vi "Fit VI window to Largest Dec__ogtk.vi"(4 "error in (no error)":errorcluster, 6 "border spacing (2 px)":i32=2, 7 "VI Ref (calling VI)":refnum<vi>) -> (0 "error out":errorcluster, 3 "dup VI Ref":refnum<vi>)   [LabVIEW 2017]
doc: "This utility will fit (resize and center) a VI (defined by the \"VI Ref\" input) about the largest decoration in that VI. It will add a border defined by border spacing in units of pixels. If there are no decorations found in the VI it is a no-op and will not produce an error. Unfortunately, this VI can not find locked decorations (yet)."
uses:
  <vilib>/Utility/miscctls.llb/LVRectTypeDef.ctl
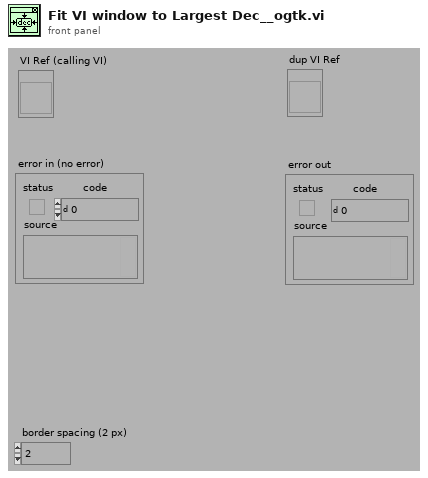
[diagram p1: front panel]
types:
  T1 = typedef "LVRectTypeDef.ctl" = cluster{"Left":i16, "Top":i16, "Right":i16, "Bottom":i16}
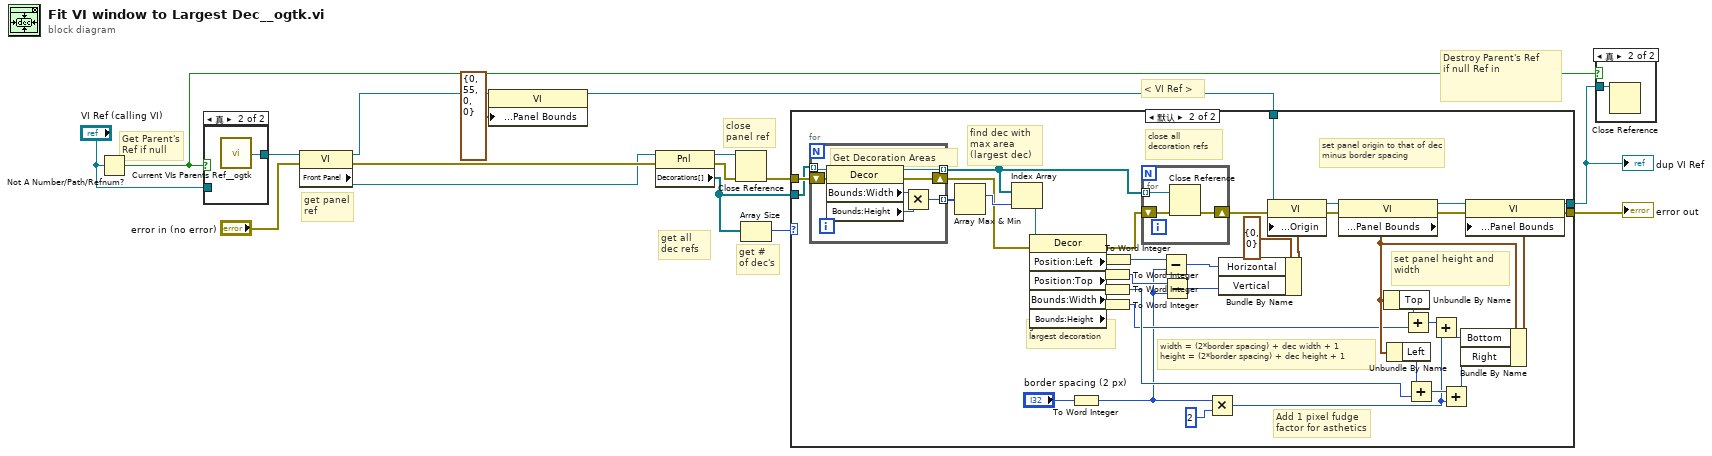
[diagram p0: block diagram]
diagram:
  # "Destroy Parent's Ref\nif null Ref in"
  # "Get Parent's\nRef if null"
  # "get # of dec's"
  # "get panel ref"
  # "get all dec refs"
  # "close panel ref"
  # "< VI Ref >"
  n1 = Not A Number/Path/Refnum?(number/path/refnum="VI Ref (calling VI)") -> (NaN/Path/Refnum?=w5:bool)
  n2 = case shown="真" w5 {
    tunnel: [w17 w18] -> w6
    tunnel: "VI Ref (calling VI)" -> [w17 _]
    frame False {
    }
    frame True {
      n3 = call "Current VIs Parents Ref__ogtk.vi"() -> ("Calling VI's reference"=w18:refnum<vi>)  [unwired: 2 in]
    }
  }
  n4 = property on="Property Node" class="VI"(reference=w6, error in="error in (no error)") -> (reference out=w3:refnum<vi>, error out=w15:errorcluster, "Front Panel"=w12:refnum<vi>)
  n5 = property on="Property Node" class="VI"(reference=w3, "Front Panel Window:Panel Bounds"=T1 {"Left"=0, "Top"=55, "Right"=0, "Bottom"=0} ("前面板窗口:前面板边界")) -> (reference out=w2:refnum<vi>)  [unwired: 1 in, 1 out]
  n6 = property on="Property Node" class="Pnl"(reference=w12, error in=w15) -> (reference out=w16:refnum<vi>, error out=w14:errorcluster, "Decorations[]"=w9:refnum<vi>[])
  n7 = Close Reference(reference=w16, error in (no error)=w14) -> (error out=w11:errorcluster)
  n8 = Array Size(array=w9) -> (size(s)=w8:i32)
  n9 = case shown="默认" w8 {
    tunnel: w2 -> [w20 w58]
    tunnel: w11 -> [w19 w41]
    tunnel: [w19 w29] -> w10
    tunnel: [w20 w28] -> w4
    tunnel: w9 -> [_ w27]
    frame 0 {
      # "do nothing if no decorations"
    }
    frame Default {
      # "width = (2*border spacing) + dec width + 1\nheight = (2*border spacing) + dec height + 1"
      # "set panel height and width"
      # "set panel origin to that of dec minus border spacing"
      # "close all  decoration refs"
      # "get coord's of largest decoration"
      # "Add 1 pixel fudge factor for asthetics"
      # "find dec with max area (largest dec)"
      n10 = for {
        tunnel: w27 -> [w67] mode=indexing
        tunnel: [w64] -> w40 mode=indexing
        shift-right: [w62] -> w36
        shift-left: w41 -> [w63]
        tunnel: [w61] -> w38 mode=indexing
        # "Get Decoration Areas"
        n11 = property class="Decor"(reference=w67, error in=w63) -> (reference out=w61:refnum<vi>, error out=w62:errorcluster, "Bounds:Width"=w66:u32, "Bounds:Height"=w65:u32)
        n12 = Multiply(x=w66, y=w65) -> (x*y=w64:u32)
      }
      n13 = Array Max & Min(array=w40) -> (max index (indices)=w39:i32)  [unwired: 3 out]
      n14 = Index Array(array=w38, index=w39) -> (element=w37:refnum<vi>)
      n15 = property class="Decor"(reference=w37, error in=w36) -> (error out=w35:errorcluster, "Position:Left"=w44:i32, "Position:Top"=w47:i32, "Bounds:Width"=w52:u32, "Bounds:Height"=w50:u32)  [unwired: 1 out]
      n16 = To Word Integer(number="border spacing (2 px)") -> (16bit integer=w21:i16)
      n17 = To Word Integer(number=w47) -> (16bit integer=w22:i16)
      n18 = To Word Integer(number=w52) -> (16bit integer=w25:i16)
      n19 = To Word Integer(number=w50) -> (16bit integer=w24:i16)
      n20 = To Word Integer(number=w44) -> (16bit integer=w23:i16)
      n21 = for {
        tunnel: w38 -> [w70] mode=indexing
        shift-right: [w68] -> w32
        shift-left: w35 -> [w69]
        n22 = Close Reference(reference=w70, error in (no error)=w69) -> (error out=w68:errorcluster)
      }
      n23 = Subtract(x=w23, y=w21) -> (x-y=w45:i16)
      n24 = Subtract(x=w22, y=w21) -> (x-y=w46:i16)
      n25 = Multiply(x=w21, y=i16 2) -> (x*y=w26:i16)
      n26 = Bundle By Name(cluster=cluster{"Horizontal":i16, "Vertical":i16} {"Horizontal"=0, "Vertical"=0} ("Front Panel Window:Origin"), "Horizontal"=w45, "Vertical"=w46) -> (w42:cluster{"Horizontal":i16, "Vertical":i16})
      n27 = property on="Property Node" class="VI"(reference=w58, error in=w32, "Front Panel Window:Origin"=w42) -> (reference out=w59:refnum<vi>, error out=w31:errorcluster)
      n28 = property on="Property Node" class="VI"(reference=w59, error in=w31) -> (reference out=w60:refnum<vi>, error out=w30:errorcluster, "Front Panel Window:Panel Bounds"=w48:T1)
      n29 = Unbundle By Name(w48) -> ("Top"=w49:i16)
      n30 = Unbundle By Name(w48) -> ("Left"=w51:i16)
      n31 = Add(x=w49, y=w24) -> (x+y=w56:i16)
      n32 = Add(x=w51, y=w25) -> (x+y=w54:i16)
      n33 = Add(x=w56, y=w26) -> (x+y=w57:i16)
      n34 = Add(x=w54, y=w26) -> (x+y=w55:i16)
      n35 = Bundle By Name(cluster=w48, "Bottom"=w57, "Right"=w55) -> (w53:T1)
      n36 = property on="Property Node" class="VI"(reference=w60, error in=w30, "Front Panel Window:Panel Bounds"=w53) -> (reference out=w28:refnum<vi>, error out=w29:errorcluster)
    }
  }
  "error out" <- w10
  "dup VI Ref" <- w4
  n37 = case shown="真" w5 {
    tunnel: w4 -> [_ w71]
    frame False {
    }
    frame True {
      n38 = Close Reference(reference=w71) -> ()  [unwired: 1 in, 1 out]
    }
  }
